vi "TDC_setExposureTime.vi"(8 "Error In":errorcluster, 11 "Exposure Time [ms]":i32 min=1) -> (0 "Error Out":errorcluster)   [LabVIEW 2011]
uses:
  dist/userlib/lib/tdcbase.dll
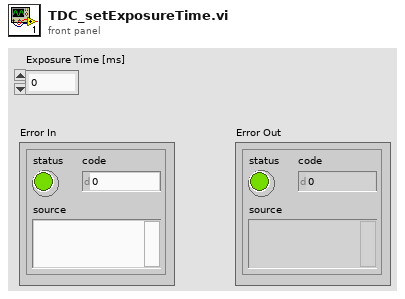
[diagram p1: front panel]
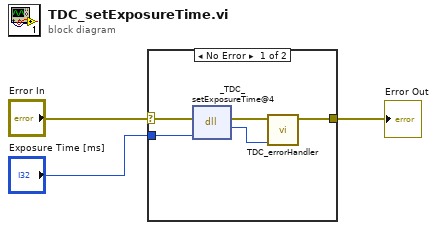
[diagram p0: block diagram]
diagram:
  n1 = case shown="No Error" "Error In" {
    selector: "Error In" -> [w7 w9]
    tunnel: [w4 w9] -> w2
    tunnel: "Exposure Time [ms]" -> [w8 _]
    frame No Error {
      n2 = dll-call lib="C:/nh/projekt/spmctrl/dist/userlib/lib/tdcbase.dll" fn="_TDC_setExposureTime@4"(error in=w7, "expTime"=w8) -> (error out=w6:errorcluster, "return type"=w5:i32)  [unwired: 3 in, 1 out]
      n3 = call "TDC_errorHandler.vi"("quTAU Return Code"=w5, "Error In"=w6) -> ("Error Out"=w4:errorcluster)  [unwired: 9 in]
    }
    frame Error {
    }
  }
  "Error Out" <- w2
